vi "Names Data Set.vi"(0 "Name Actions":T1, 11 "error in (no error)":errorcluster) -> (1 "Actuator Command Volts":string[](array[string])=["Actuator Command X1 (V)", "Actuator Command X2 (V)", "Actuator Command Y1 (V)", "Actuator Command Z1 (V)", "Actuator Command Z2 (V)", "Actuator Command Z3 (V)"], 2 "Actuator Volt Readings":string[](array[string])=["Actuator LVDT X1 (V)", "Actuator LVDT X2 (V)", "Actuator LVDT Y1 (V)", "Actuator LVDT Z1 (V)", "Actuator LVDT Z2 (V)", "Actuator LVDT Z3 (V)", "Actuator LC X1 (V)", "Actuator LC X2 (V)", "Actuator LC Y1 (V)", "Actuator LC Z1 (V)", "Actuator LC Z2 (V)", "Actuator LC Z3 (V)"], 3 "Servo Names":string[](array[string])=["Servo Error X1 (V)", "Servo Error X2 (V)", "Servo Error Y1 (V)", "Servo Error Z1 (V)", "Servo Error Z2 (V)", "Servo Error Z3 (V)"], 4 "Cartesian Commands":string[](array[string])=["Cartesian Command X (in)", "Cartesian Command Y (in)", "Cartesian Command Z (in)", "Cartesian Command Rx (rad)", "Cartesian Command Ry (rad)", "Cartesian Command Rz (rad)"], 6 "Cartesian Readings":string[](array[string])=["Cartesian X (in)", "Cartesian Y (in)", "Cartesian Z (in)", "Cartesian Rx (rad)", "Cartesian Ry (rad)", "Cartesian Rz (rad)", "Cartesian Fx (lb)", "Cartesian Fy (lb)", "Cartesian Fz (lb)", "Cartesian Mx (lb*in)", "Cartesian My (lb*in)", "Cartesian Mz (lb*in)"], 8 "Actuator Commands":string[](array[string])=["Actuator Command X1 (in)", "Actuator Command X2 (in)", "Actuator Command Y1 (in)", "Actuator Command Z1 (in)", "Actuator Command Z2 (in)", "Actuator Command Z3 (in)"], 10 "Actuator Readings":string[](array[string])=["Actuator Stroke X1 (in)", "Actuator Stroke X2 (in)", "Actuator Stroke Y1 (in)", "Actuator Stroke Z1 (in)", "Actuator Stroke Z2 (in)", "Actuator Stroke Z3 (in)", "Actuator Force X1 (lb)", "Actuator Force X2 (lb)", "Actuator Force Y1 (lb)", "Actuator Force Z1 (lb)", "Actuator Force Z2 (lb)", "Actuator Force Z3 (lb)"], 13 "External Sensor Names":string[](array[string]), 14 "Cartesian Force Commands":string[](array[string])=["Cartesian Command Fx (lb)", "Cartesian Command Fy (lb)", "Cartesian Command Fz (lb)", "Cartesian Command Mx (lb*in)", "Cartesian Command My (lb*in)", "Cartesian Command Mz (lb*in)"], 15 "error out":errorcluster)   [LabVIEW 2009]
uses:
  Names/Name Actions.ctl
  Data Access Objects/Metadata/LBCB Number.ctl
  Data Access Objects/Metadata/Persistant DAO Actions.ctl
panel:
  in  "Actuators":string[](array[string])=[" X1", " X2", " Y1", " Z1", " Z2", " Z3"]
  in  "Cartesian Force":string[](array[string])=[" Fx (lbs)", " Fy (lbs)", " Fz (lbs)", " Mx (lb*in)", " My (lb*in)", " Mz (lb*in)"]
  in  "Cartesian Displacement Units":string[](array[string])=[" X (in)", " Y (in)", " Z (in)", " Rx (rad)", " Ry (rad)", " Rz (rad)"]
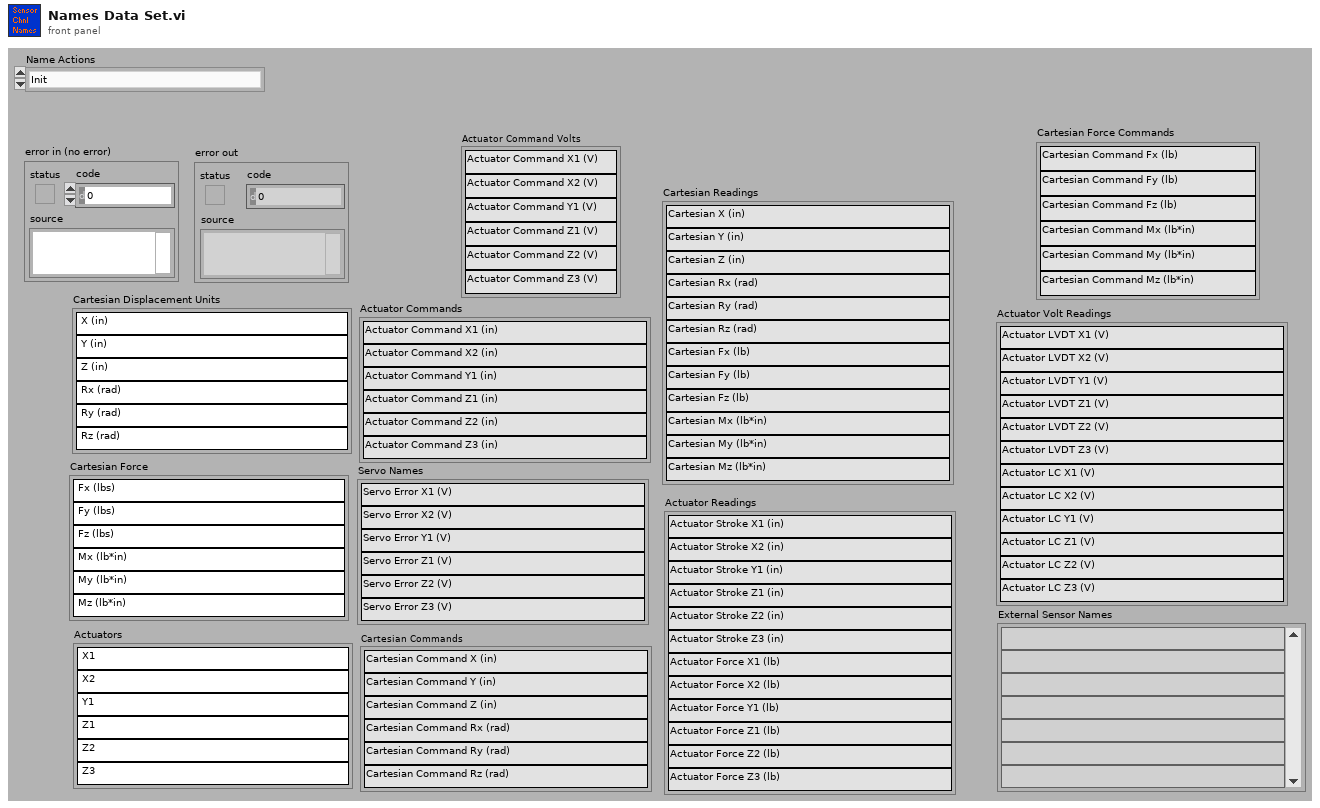
[diagram p1: front panel]
types:
  T1 = typedef "Name Actions.ctl" = enum16{"Init", "Get Names", "Get Index"}
  T2 = typedef "LBCB Number.ctl" = enum16{"LBCB1", "LBCB2"}
  T3 = typedef "Persistant DAO Actions.ctl" = enum16{"Init", "Get", "Set", "Load", "Save"}
  T4 = typedef "LBCB Settings.ctl" = cluster{"Size":T5, "Type":T6}
  T5 = typedef "LBCB Size.ctl" = enum16{"1/5th-scale LBCB", "Full-scale LBCB", "Portable LBCB"}
  T6 = typedef "LBCB Type.ctl" = enum16{"X Actuators On The Left", "X Actuators On The Right"}
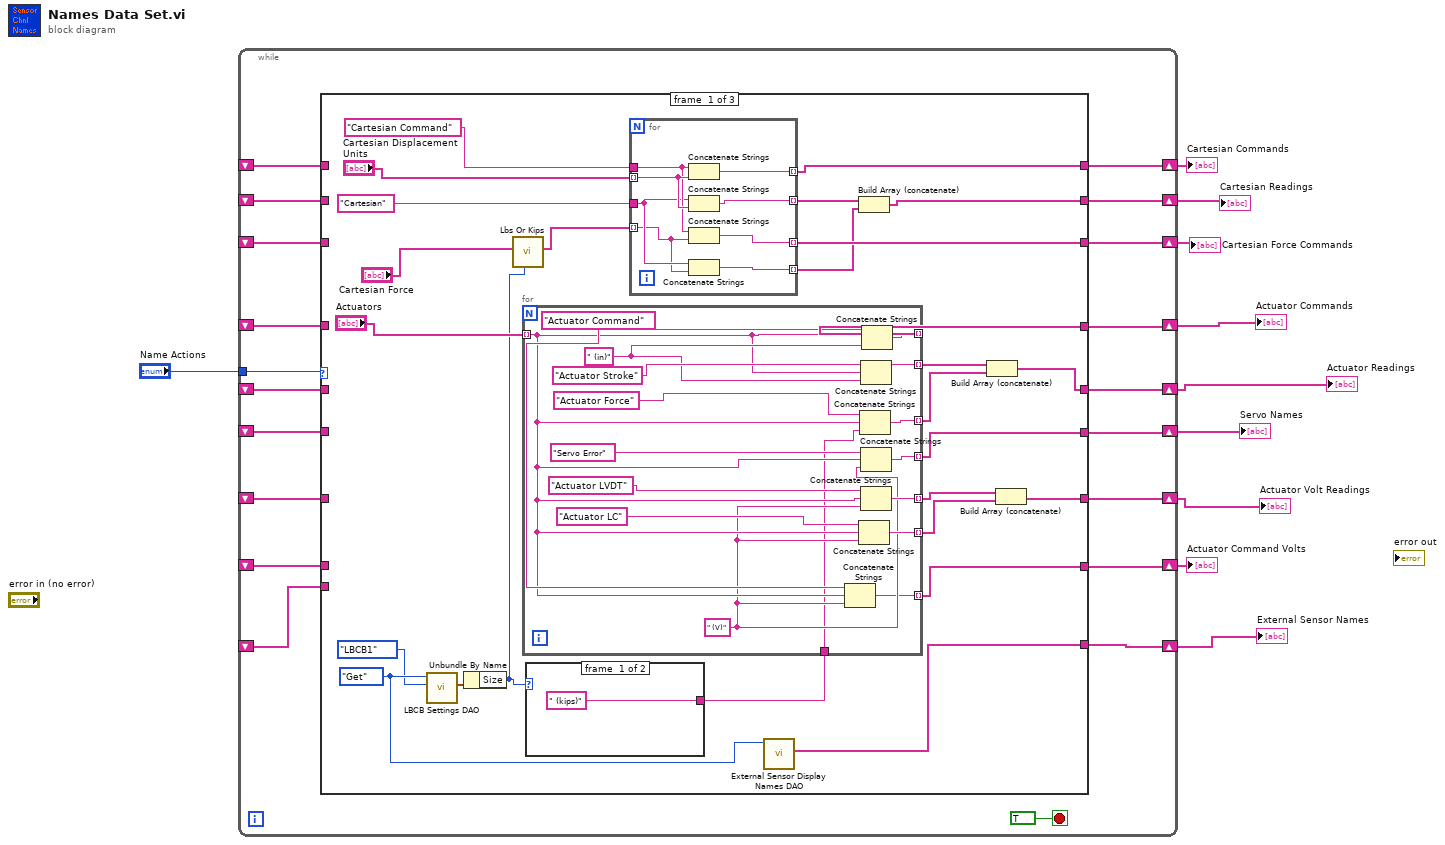
[diagram p0: block diagram]
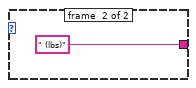
[diagram p2: hidden frame]
diagram:
  n1 = while {
    tunnel: "Name Actions" -> [w29]
    shift-right: [w28] -> w9
    shift-left: _ -> [w24]
    shift-right: [w27] -> w8
    shift-left: _ -> [w22]
    shift-right: [w26] -> w7
    shift-left: _ -> [w23]
    shift-right: [w25] -> w6
    shift-left: _ -> [w21]
    shift-right: [w20] -> w5
    shift-left: _ -> [w19]
    shift-right: [w18] -> w4
    shift-left: _ -> [w17]
    shift-right: [w16] -> w3
    shift-left: _ -> [w15]
    shift-right: [w14] -> w2
    shift-left: _ -> [w13]
    shift-right: [w12] -> w1
    shift-left: _ -> [w11]
    stop <- TRUE stop-if-true
    n2 = case shown="\"Init\"" w29 {
      tunnel: [w47 w92 w101] -> w28
      tunnel: [w42 w90 w99] -> w27
      tunnel: [w41 w91 w100] -> w26
      tunnel: [w40 w89 w98] -> w25
      tunnel: w24 -> [_ w92 w101]
      tunnel: w23 -> [_ w91 w100]
      tunnel: w22 -> [_ w90 w99]
      tunnel: w21 -> [_ w89 w98]
      tunnel: [w46 w88 w97] -> w20
      tunnel: w19 -> [_ w88 w97]
      tunnel: [w44 w87 w96] -> w18
      tunnel: w17 -> [_ w87 w96]
      tunnel: [w45 w86 w95] -> w16
      tunnel: w15 -> [_ w86 w95]
      tunnel: [w43 w85 w94] -> w14
      tunnel: w13 -> [_ w85 w94]
      tunnel: [w39 w84 w93] -> w12
      tunnel: w11 -> [_ w84 w93]
      frame #0 {
        w37 = Persistant_DAO_Actions."Get" ("Persistent DAO Actions")
        n3 = call "LBCB Settings DAO.vi"("LBCB Number"=LBCB_Number."LBCB1", "Actions"=w37) -> ("LBCB Setting Out"=w35:T4)  [unwired: 7 in, 2 out]
        n4 = Unbundle By Name(w35) -> ("Size"=w31:T5)
        n5 = call "Lbs Or Kips.vi"("Size"=w31, "Cartesian Force In"="Cartesian Force") -> ("Cartesian Force In Out"=w32:string[])  [unwired: 9 in]
        n6 = case shown="\"Full-scale LBCB\"" w31 {
          tunnel: [" (kips)" ("string") " (lbs)" ("string")] -> w34
          frame #0 {
          }
          frame #1 {
          }
        }
        n7 = for {
          tunnel: "Actuators" -> [w62] mode=indexing
          tunnel: [w69] -> w44 mode=indexing
          tunnel: [w68] -> w51 mode=indexing
          tunnel: [w67] -> w50 mode=indexing
          tunnel: [w66] -> w41 mode=indexing
          tunnel: [w65] -> w49 mode=indexing
          tunnel: [w64] -> w48 mode=indexing
          tunnel: [w60] -> w43 mode=indexing
          tunnel: w34 -> [w59]
          w61 = " (V)" ("string")
          w74 = " (in)" ("string")
          w63 = "Actuator Command" ("string")
          n8 = Concatenate Strings(w63, w62, w61) -> (w60:string)
          n9 = Concatenate Strings("Actuator LC" ("string"), w62, w61) -> (w64:string)
          n10 = Concatenate Strings("Actuator Force" ("string"), w62, w59) -> (w67:string)
          n11 = Concatenate Strings("Actuator Stroke" ("string"), w62, w74) -> (w68:string)
          n12 = Concatenate Strings("Servo Error" ("string"), w62, w61) -> (w66:string)
          n13 = Concatenate Strings("Actuator LVDT" ("string"), w62, w61) -> (w65:string)
          n14 = Concatenate Strings(w63, w62, w74) -> (w69:string)
        }
        n15 = for {
          tunnel: "Cartesian Command" ("string") -> [w80]
          tunnel: "Cartesian Displacement Units" -> [w82] mode=indexing
          tunnel: "Cartesian" ("string") -> [w78]
          tunnel: [w83] -> w45 mode=indexing
          tunnel: [w81] -> w53 mode=indexing
          tunnel: w32 -> [w77] mode=indexing
          tunnel: [w79] -> w39 mode=indexing
          tunnel: [w76] -> w38 mode=indexing
          n16 = Concatenate Strings(w80, w82) -> (w83:string)
          n17 = Concatenate Strings(w78, w82) -> (w81:string)
          n18 = Concatenate Strings(w80, w77) -> (w79:string)
          n19 = Concatenate Strings(w78, w77) -> (w76:string)
        }
        n20 = call "External Sensor Display Names DAO.vi"("Persistent DAO Actions"=w37) -> ("Display Name Out"=w40:string[])  [unwired: 3 in, 7 out]
        n21 = Build Array (concatenate)(w53, w38) -> (w47:string[])
        n22 = Build Array (concatenate)(w51, w50) -> (w46:string[])
        n23 = Build Array (concatenate)(w49, w48) -> (w42:string[])
      }
      frame #1 {
      }
      frame #2 {
      }
    }
  }
  "Cartesian Readings" <- w9
  "Actuator Volt Readings" <- w8
  "Servo Names" <- w7
  "External Sensor Names" <- w6
  "Actuator Readings" <- w5
  "Actuator Commands" <- w4
  "Cartesian Commands" <- w3
  "Actuator Command Volts" <- w2
  "Cartesian Force Commands" <- w1
